vi "Exit Windows Ex.vi"(8 "error in (no error)":errorcluster, 10 "dwReserved":u32, 11 "uFlags":u32) -> (0 "error out":errorcluster, 3 "return type":i32)   [LabVIEW 2020, in "QCT ALARM.lvlib"]
uses:
  QCT ALARM.lvlib
  Windows/System32/user32.dll
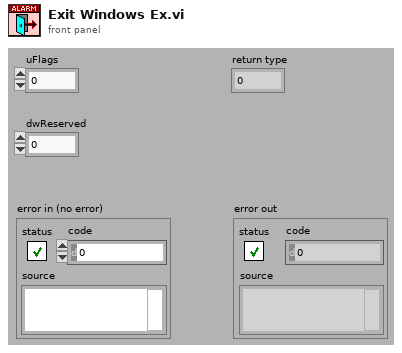
[diagram p1: front panel]
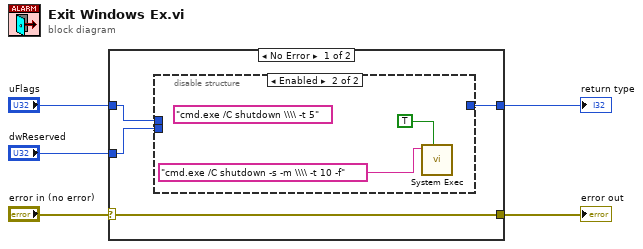
[diagram p0: block diagram]
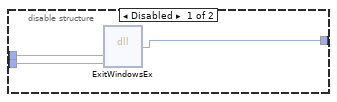
[diagram p2: hidden frame]
diagram:
  n1 = case shown="No Error" "error in (no error)" {
    selector: "error in (no error)" -> [w9 w15]
    tunnel: [w9 w15] -> w4
    tunnel: [w8 _] -> w3
    tunnel: "uFlags" -> [w7 _]
    tunnel: "dwReserved" -> [w6 _]
    frame No Error {
      n2 = disable-structure shown="Enabled" {
        disable-tunnel: [w12 _] -> w8
        disable-tunnel: w7 -> [w11 _]
        disable-tunnel: w6 -> [w10 _]
        frame Disabled {
          n3 = dll-call lib="/Windows/System32/user32.dll" fn="ExitWindowsEx"("uFlags"=w11, "dwReserved"=w10) -> ("return type"=w12:i32)  [unwired: 5 in, 2 out]
        }
        frame Enabled {
          (unwired) "cmd.exe /C shutdown \\\\ -t 5"
          n4 = call <vilib>:"System Exec.vi"("wait until completion? (T)"=TRUE, "command line"="cmd.exe /C shutdown -s -m \\\\ -t 10 -f") -> ()  [unwired: 6 in, 4 out]
        }
      }
    }
    frame Error {
    }
  }
  "return type" <- w3
  "error out" <- w4
